vi "InitGlobalPreferences.vi"(8 "error in (no error)":errorcluster, 11 "Preferences in":refnum<class "SetListPrefs.lvclass">) -> (0 "error out":errorcluster, 2 "Raw XML":string, 3 "Preferences out":refnum<class "SetListPrefs.lvclass">)   [LabVIEW 2013, in "SetListPrefs.lvclass"]
uses:
  SetListPrefs.lvclass
  Globals/PrefsGlobal.vi
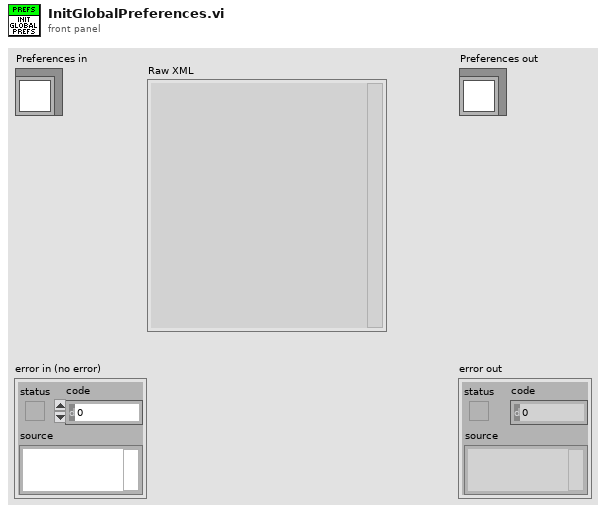
[diagram p1: front panel]
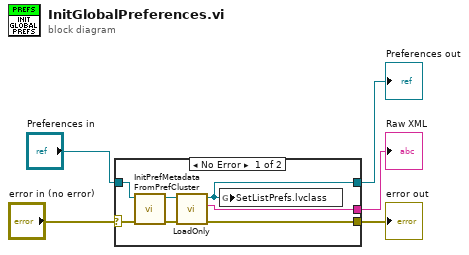
[diagram p0: block diagram]
diagram:
  n1 = case shown="No Error" "error in (no error)" {
    selector: "error in (no error)" -> [w11 w14]
    tunnel: [w7 w14] -> w4
    tunnel: [w6 w13] -> w2
    tunnel: "Preferences in" -> [w12 w13]
    tunnel: [w8 _] -> w1
    frame No Error {
      n2 = call "InitPrefMetadataFromPrefCluster.vi"("error in (no error)"=w11, "Preferences in"=w12) -> ("error out"=w10:errorcluster, "Preferences out"=w9:refnum<class "SetListPrefs.lvclass">)  [unwired: 8 in]
      n3 = call "LoadOnly.vi"("error in (no error)"=w10, "Preferences in"=w9) -> ("error out"=w7:errorcluster, "Raw XML"=w8:string, "Preferences out"=w6:refnum<class "SetListPrefs.lvclass">)  [unwired: 7 in]
      n4 = global write "PrefsGlobal.vi" "SetListPrefs.lvclass"(w6) -> ()
    }
    frame Error {
    }
  }
  "error out" <- w4
  "Preferences out" <- w2
  "Raw XML" <- w1
